vi "CRUD Update Example.vi"() -> ()   [LabVIEW 2020, in "ORM_Examples.lvlib"]
doc: "This will update the row specified by the primary key value \"pNum\" using the values for the private data of bbPlayers provided as inputs. Note that BB Players Map is also used."
uses:
  ORM_Examples.lvlib
  BB Players Map/BB Players Map.lvclass
  C:/Program Files/National Instruments/LabVIEW 2020/vi.lib/Viviota/shared/ORM.lvlibp/ORM/TypeMap/TypeMap.lvclass
  C:/Program Files/National Instruments/LabVIEW 2020/vi.lib/Viviota/shared/ORM.lvlibp/Transaction Logger/Log Map/LogMap.lvclass
  BB Players/bbPlayers.lvclass
  22d36fc3-13e9-48d3-82bb-267a5c78aea6.vi
  22d36fc3-13e9-48d3-82bb-267a5c78aea6.vi/bf74eca6-e633-4dc5-891a-edef426d4fd9.vi
  <vilib>/Viviota/shared/ORM_ADONet.lvlibp/ADOMapper/ADOMapper.lvclass
  C:/Program Files/National Instruments/LabVIEW 2020/vi.lib/Viviota/shared/ORM.lvlibp/ORM/SqlMapper/SqlMapper.lvclass
  <vilib>/Viviota/shared/ORM.lvlibp/ORM/TypeMap/Write Autokey.vi
  <vilib>/Viviota/shared/ORM.lvlibp/ORM/TypeMap/Write Table Name.vi
  <vilib>/Viviota/shared/ORM.lvlibp/Transaction Logger/Log Map/Write Log Table Name.vi
  <vilib>/Viviota/shared/ORM_DBC_Sqlite.lvlibp/Sqlite Connect.vi
  <vilib>/Utility/error.llb/Error Cluster From Error Code.vi
  <vilib>/Viviota/shared/ORM.lvlibp/ORM/TypeMap/Read TypeMap.vi
  <vilib>/Viviota/shared/ORM.lvlibp/ORM/SqlMapper/End Transaction.vi
  <vilib>/Viviota/shared/ORM.lvlibp/ORM/TypeMap/TypeMap.lvclass
  ORM_API/ORM_API.lvlib
  <vilib>/Viviota/shared/ORM_ADONet.lvlibp
  <vilib>/Viviota/shared/ORM_DBC_Sqlite.lvlibp/DBC.lvclass
  C:/Program Files/National Instruments/LabVIEW 2020/vi.lib/Viviota/shared/ORM_ADONet.lvlibp/ADOMapper/ADOMapper.lvclass
panel:
  in  "pNum":i32
  in  "pAvailable":bool
  in  "pAverage":dbl
  in  "pGames":i32
  in  "pName":string
  out "affectedRows":i32
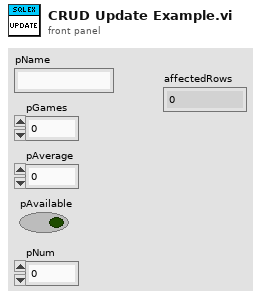
[diagram p1: front panel]
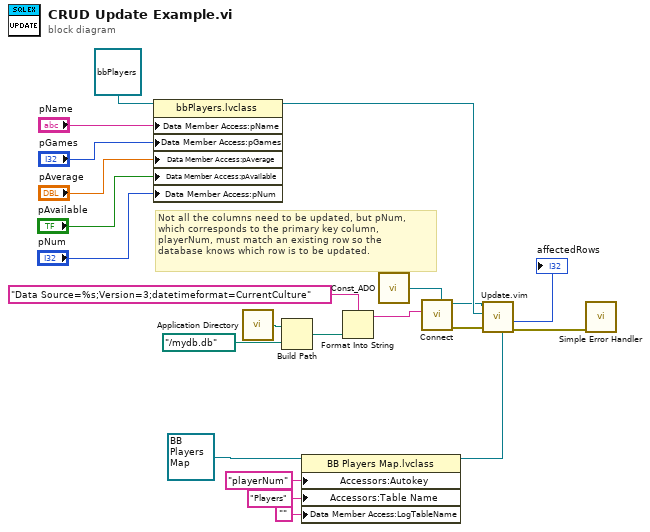
[diagram p0: block diagram]
diagram:
  # "Not all the columns need to be updated, but pNum, \nwhich corresponds to the primary key column,\nplayerNum, must match an existing row so the \ndatabase knows which row is to be updated."
  n1 = property class="bbPlayers.lvclass"(reference=refnum<class "bbPlayers.lvclass"> refnum ("bbPlayers.lvclass"), "Data Member Access:pName"="pName", "Data Member Access:pGames"="pGames", "Data Member Access:pAverage"="pAverage", "Data Member Access:pAvailable"="pAvailable", "Data Member Access:pNum"="pNum") -> (reference out=w14:refnum<class "bbPlayers.lvclass">)  [unwired: 1 in, 1 out]
  n2 = call <vilib>:"Application Directory.vi"() -> ("Application Directory"=w7:path)
  n3 = Build Path(base path=w7, name or relative path=path "../mydb.db" ("file out")) -> (appended path=w8:path)
  n4 = property class="BB Players Map.lvclass"(reference=refnum<class "BB Players Map.lvclass"> refnum ("BB Players Map.lvclass"), "Accessors:Autokey"="playerNum" ("Autokey"), "Accessors:Table Name"="Players" ("Table Name"), "Data Member Access:LogTableName"="") -> (reference out=w16:refnum<class "BB Players Map.lvclass">)  [unwired: 1 in, 1 out]
  n5 = Format Into String(format string="Data Source=%s;Version=3;datetimeformat=CurrentCulture" ("connectionStringName"), w8) -> (resulting string=w3:string)  [unwired: 2 in, 1 out]
  n6 = call <vilib>:"Const_ADO.vi"() -> ("ADOMapper"=w4:refnum<class "ADOMapper.lvclass">)
  n7 = call-poly "Connect.vi"("SqlMapper Type"=w4, "Connection String"=w3) -> ("error out"=w1:errorcluster, "SqlMapper out"=w2:refnum<class "ADOMapper.lvclass">)  [unwired: 8 in]
  n8 = call "Update.vim"("TypeMap in"=w16, "error in (no error)"=w1, "object in"=w14, "SqlMapper in"=w2) -> ("error out"=w22:errorcluster, "affectedRows"=→"affectedRows":i32)  [unwired: 4 in, 2 out]
  n9 = call <vilib>:"Simple Error Handler.vi"("error in (no error)"=w22) -> ()  [unwired: 4 in, 5 out]
